vi "Flow Array Compare.vi"(10 "Flow Array in":dbl[](array[numeric]), 11 "Array in":dbl[](array[numeric])) -> (3 "Array out":dbl[](array[numeric]))   [LabVIEW 2020, in "CollectionSupport.lvlib"]
uses:
  CollectionSupport.lvlib
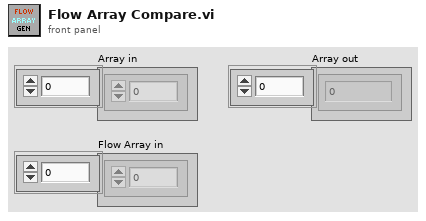
[diagram p1: front panel]
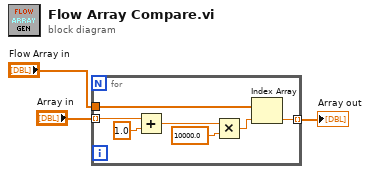
[diagram p0: block diagram]
diagram:
  n1 = for {
    tunnel: "Array in" -> [w6] mode=indexing
    tunnel: "Flow Array in" -> [w10]
    tunnel: [w7] -> w3 mode=indexing
    n2 = Add(x=w6, y=1.0) -> (x+y=w5:dbl)
    n3 = Multiply(x=w5, y=10000.0) -> (x*y=w8:dbl)
    n4 = Index Array(array=w10, index=w8) -> (element=w7:dbl)
  }
  "Array out" <- w3
